vi "DDS_Clock.vi"() -> ()   [LabVIEW 2016] (continued)
{"total time[ms]"=60.64999999999869, "f1 [Hz] CH0"=302600000.00000006}, {"total time[ms]"=60.69999999999869, "f1 [Hz] CH0"=302800000.0}, {"total time[ms]"=60.69999999999869, "f1 [Hz] CH0"=302800000.0}, {"total time[ms]"=60.749999999998685, "f1 [Hz] CH0"=303000000.0}, {"total time[ms]"=60.749999999998685, "f1 [Hz] CH0"=303000000.0}, {"total time[ms]"=60.79999999999868, "f1 [Hz] CH0"=303200000.00000006}, {"total time[ms]"=60.79999999999868, "f1 [Hz] CH0"=303200000.00000006}, {"total time[ms]"=60.84999999999868, "f1 [Hz] CH0"=303400000.00000006}, {"total time[ms]"=60.84999999999868, "f1 [Hz] CH0"=303400000.00000006}, {"total time[ms]"=60.89999999999868, "f1 [Hz] CH0"=303600000.0}, {"total time[ms]"=60.89999999999868, "f1 [Hz] CH0"=303600000.0}, {"total time[ms]"=60.949999999998674, "f1 [Hz] CH0"=303800000.0}, {"total time[ms]"=60.949999999998674, "f1 [Hz] CH0"=303800000.0}, {"total time[ms]"=60.99999999999867, "f1 [Hz] CH0"=304000000.0}, {"total time[ms]"=60.99999999999867, "f1 [Hz] CH0"=304000000.0}, {"total time[ms]"=61.04999999999867, "f1 [Hz] CH0"=304200000.0}, {"total time[ms]"=61.04999999999867, "f1 [Hz] CH0"=304200000.0}, {"total time[ms]"=61.099999999998666, "f1 [Hz] CH0"=304400000.0}, {"total time[ms]"=61.099999999998666, "f1 [Hz] CH0"=304400000.0}, {"total time[ms]"=61.14999999999866, "f1 [Hz] CH0"=304600000.00000006}, {"total time[ms]"=61.14999999999866, "f1 [Hz] CH0"=304600000.00000006}, {"total time[ms]"=61.19999999999866, "f1 [Hz] CH0"=304800000.00000006}, {"total time[ms]"=61.19999999999866, "f1 [Hz] CH0"=304800000.00000006}, {"total time[ms]"=61.24999999999866, "f1 [Hz] CH0"=305000000.0}, {"total time[ms]"=61.24999999999866, "f1 [Hz] CH0"=305000000.0}, {"total time[ms]"=61.299999999998654, "f1 [Hz] CH0"=305200000.00000006}, {"total time[ms]"=61.299999999998654, "f1 [Hz] CH0"=305200000.00000006}, {"total time[ms]"=61.34999999999865, "f1 [Hz] CH0"=305400000.0}, {"total time[ms]"=61.34999999999865, "f1 [Hz] CH0"=305400000.0}, {"total time[ms]"=61.39999999999865, "f1 [Hz] CH0"=305600000.0}, {"total time[ms]"=61.39999999999865, "f1 [Hz] CH0"=305600000.0}, {"total time[ms]"=61.449999999998646, "f1 [Hz] CH0"=305800000.0}, {"total time[ms]"=61.449999999998646, "f1 [Hz] CH0"=305800000.0}, {"total time[ms]"=61.49999999999864, "f1 [Hz] CH0"=306000000.0}, {"total time[ms]"=61.49999999999864, "f1 [Hz] CH0"=306000000.0}, {"total time[ms]"=61.54999999999864, "f1 [Hz] CH0"=306200000.00000006}, {"total time[ms]"=61.54999999999864, "f1 [Hz] CH0"=306200000.00000006}, {"total time[ms]"=61.59999999999864, "f1 [Hz] CH0"=306400000.0}, {"total time[ms]"=61.59999999999864, "f1 [Hz] CH0"=306400000.0}, {"total time[ms]"=61.649999999998634, "f1 [Hz] CH0"=306600000.00000006}, {"total time[ms]"=61.649999999998634, "f1 [Hz] CH0"=306600000.00000006}, {"total time[ms]"=61.69999999999863, "f1 [Hz] CH0"=306800000.00000006}, {"total time[ms]"=61.69999999999863, "f1 [Hz] CH0"=306800000.00000006}, {"total time[ms]"=61.74999999999863, "f1 [Hz] CH0"=307000000.0}, {"total time[ms]"=61.74999999999863, "f1 [Hz] CH0"=307000000.0}, {"total time[ms]"=61.799999999998626, "f1 [Hz] CH0"=307200000.0}, {"total time[ms]"=61.799999999998626, "f1 [Hz] CH0"=307200000.0}, {"total time[ms]"=61.84999999999862, "f1 [Hz] CH0"=307400000.0}, {"total time[ms]"=61.84999999999862, "f1 [Hz] CH0"=307400000.0}, {"total time[ms]"=61.89999999999862, "f1 [Hz] CH0"=307600000.00000006}, {"total time[ms]"=61.89999999999862, "f1 [Hz] CH0"=307600000.00000006}, {"total time[ms]"=61.94999999999862, "f1 [Hz] CH0"=307800000.0}, {"total time[ms]"=61.94999999999862, "f1 [Hz] CH0"=307800000.0}, {"total time[ms]"=61.999999999998614, "f1 [Hz] CH0"=308000000.0}, {"total time[ms]"=61.999999999998614, "f1 [Hz] CH0"=308000000.0}, {"total time[ms]"=62.04999999999861, "f1 [Hz] CH0"=308200000.00000006}, {"total time[ms]"=62.04999999999861, "f1 [Hz] CH0"=308200000.00000006}, {"total time[ms]"=62.09999999999861, "f1 [Hz] CH0"=308400000.00000006}, {"total time[ms]"=62.09999999999861, "f1 [Hz] CH0"=308400000.00000006}, {"total time[ms]"=62.149999999998606, "f1 [Hz] CH0"=308600000.0}, {"total time[ms]"=62.149999999998606, "f1 [Hz] CH0"=308600000.0}, {"total time[ms]"=62.1999999999986, "f1 [Hz] CH0"=308800000.0}, {"total time[ms]"=62.1999999999986, "f1 [Hz] CH0"=308800000.0}, {"total time[ms]"=62.2499999999986, "f1 [Hz] CH0"=309000000.0}, {"total time[ms]"=62.2499999999986, "f1 [Hz] CH0"=309000000.0}, {"total time[ms]"=62.2999999999986, "f1 [Hz] CH0"=309200000.0}, {"total time[ms]"=62.2999999999986, "f1 [Hz] CH0"=309200000.0}, {"total time[ms]"=62.349999999998595, "f1 [Hz] CH0"=309400000.0}, {"total time[ms]"=62.349999999998595, "f1 [Hz] CH0"=309400000.0}, {"total time[ms]"=62.39999999999859, "f1 [Hz] CH0"=309600000.00000006}, {"total time[ms]"=62.39999999999859, "f1 [Hz] CH0"=309600000.00000006}, {"total time[ms]"=62.44999999999859, "f1 [Hz] CH0"=309800000.00000006}, {"total time[ms]"=62.44999999999859, "f1 [Hz] CH0"=309800000.00000006}, {"total time[ms]"=62.499999999998586, "f1 [Hz] CH0"=310000000.0}, {"total time[ms]"=62.499999999998586, "f1 [Hz] CH0"=310000000.0}, {"total time[ms]"=62.54999999999858, "f1 [Hz] CH0"=310200000.00000006}, {"total time[ms]"=62.54999999999858, "f1 [Hz] CH0"=310200000.00000006}, {"total time[ms]"=62.59999999999858, "f1 [Hz] CH0"=310400000.0}, {"total time[ms]"=62.59999999999858, "f1 [Hz] CH0"=310400000.0}, {"total time[ms]"=62.64999999999858, "f1 [Hz] CH0"=310600000.0}, {"total time[ms]"=62.64999999999858, "f1 [Hz] CH0"=310600000.0}, {"total time[ms]"=62.699999999998575, "f1 [Hz] CH0"=310800000.0}, {"total time[ms]"=62.699999999998575, "f1 [Hz] CH0"=310800000.0}, {"total time[ms]"=62.74999999999857, "f1 [Hz] CH0"=311000000.0}, {"total time[ms]"=62.74999999999857, "f1 [Hz] CH0"=311000000.0}, {"total time[ms]"=62.79999999999857, "f1 [Hz] CH0"=311200000.00000006}, {"total time[ms]"=62.79999999999857, "f1 [Hz] CH0"=311200000.00000006}, {"total time[ms]"=62.849999999998566, "f1 [Hz] CH0"=311400000.0}, {"total time[ms]"=62.849999999998566, "f1 [Hz] CH0"=311400000.0}, {"total time[ms]"=62.89999999999856, "f1 [Hz] CH0"=311600000.00000006}, {"total time[ms]"=62.89999999999856, "f1 [Hz] CH0"=311600000.00000006}, {"total time[ms]"=62.94999999999856, "f1 [Hz] CH0"=311800000.00000006}, {"total time[ms]"=62.94999999999856, "f1 [Hz] CH0"=311800000.00000006}, {"total time[ms]"=62.99999999999856, "f1 [Hz] CH0"=312000000.0}, {"total time[ms]"=62.99999999999856, "f1 [Hz] CH0"=312000000.0}, {"total time[ms]"=63.049999999998555, "f1 [Hz] CH0"=312200000.0}, {"total time[ms]"=63.049999999998555, "f1 [Hz] CH0"=312200000.0}, {"total time[ms]"=63.09999999999855, "f1 [Hz] CH0"=312400000.0}, {"total time[ms]"=63.09999999999855, "f1 [Hz] CH0"=312400000.0}, {"total time[ms]"=63.14999999999855, "f1 [Hz] CH0"=312600000.00000006}, {"total time[ms]"=63.14999999999855, "f1 [Hz] CH0"=312600000.00000006}, {"total time[ms]"=63.199999999998546, "f1 [Hz] CH0"=312800000.0}, {"total time[ms]"=63.199999999998546, "f1 [Hz] CH0"=312800000.0}, {"total time[ms]"=63.24999999999854, "f1 [Hz] CH0"=313000000.0}, {"total time[ms]"=63.24999999999854, "f1 [Hz] CH0"=313000000.0}, {"total time[ms]"=63.29999999999854, "f1 [Hz] CH0"=313200000.00000006}, {"total time[ms]"=63.29999999999854, "f1 [Hz] CH0"=313200000.00000006}, {"total time[ms]"=63.34999999999854, "f1 [Hz] CH0"=313400000.00000006}, {"total time[ms]"=63.34999999999854, "f1 [Hz] CH0"=313400000.00000006}, {"total time[ms]"=63.399999999998535, "f1 [Hz] CH0"=313600000.0}, {"total time[ms]"=63.399999999998535, "f1 [Hz] CH0"=313600000.0}, {"total time[ms]"=63.44999999999853, "f1 [Hz] CH0"=313800000.0}, {"total time[ms]"=63.44999999999853, "f1 [Hz] CH0"=313800000.0}, {"total time[ms]"=63.49999999999853, "f1 [Hz] CH0"=314000000.0}, {"total time[ms]"=63.49999999999853, "f1 [Hz] CH0"=314000000.0}, {"total time[ms]"=63.549999999998526, "f1 [Hz] CH0"=314200000.0}, {"total time[ms]"=63.549999999998526, "f1 [Hz] CH0"=314200000.0}, {"total time[ms]"=63.59999999999852, "f1 [Hz] CH0"=314400000.0}, {"total time[ms]"=63.59999999999852, "f1 [Hz] CH0"=314400000.0}, {"total time[ms]"=63.64999999999852, "f1 [Hz] CH0"=314600000.00000006}, {"total time[ms]"=63.64999999999852, "f1 [Hz] CH0"=314600000.00000006}, {"total time[ms]"=63.69999999999852, "f1 [Hz] CH0"=314800000.00000006}, {"total time[ms]"=63.69999999999852, "f1 [Hz] CH0"=314800000.00000006}, {"total time[ms]"=63.749999999998515, "f1 [Hz] CH0"=315000000.0}, {"total time[ms]"=63.749999999998515, "f1 [Hz] CH0"=315000000.0}, {"total time[ms]"=63.79999999999851, "f1 [Hz] CH0"=315200000.00000006}, {"total time[ms]"=63.79999999999851, "f1 [Hz] CH0"=315200000.00000006}, {"total time[ms]"=63.84999999999851, "f1 [Hz] CH0"=315400000.0}, {"total time[ms]"=63.84999999999851, "f1 [Hz] CH0"=315400000.0}, {"total time[ms]"=63.899999999998506, "f1 [Hz] CH0"=315600000.0}, {"total time[ms]"=63.899999999998506, "f1 [Hz] CH0"=315600000.0}, {"total time[ms]"=63.949999999998504, "f1 [Hz] CH0"=315800000.0}, {"total time[ms]"=63.949999999998504, "f1 [Hz] CH0"=315800000.0}, {"total time[ms]"=63.9999999999985, "f1 [Hz] CH0"=316000000.0}, {"total time[ms]"=63.9999999999985, "f1 [Hz] CH0"=316000000.0}, {"total time[ms]"=64.0499999999985, "f1 [Hz] CH0"=316200000.0}, {"total time[ms]"=64.0499999999985, "f1 [Hz] CH0"=316200000.0}, {"total time[ms]"=64.0999999999985, "f1 [Hz] CH0"=316400000.00000006}, {"total time[ms]"=64.0999999999985, "f1 [Hz] CH0"=316400000.00000006}, {"total time[ms]"=64.1499999999985, "f1 [Hz] CH0"=316600000.00000006}, {"total time[ms]"=64.1499999999985, "f1 [Hz] CH0"=316600000.00000006}, {"total time[ms]"=64.1999999999985, "f1 [Hz] CH0"=316800000.00000006}, {"total time[ms]"=64.1999999999985, "f1 [Hz] CH0"=316800000.00000006}, {"total time[ms]"=64.2499999999985, "f1 [Hz] CH0"=317000000.0}, {"total time[ms]"=64.2499999999985, "f1 [Hz] CH0"=317000000.0}, {"total time[ms]"=64.29999999999849, "f1 [Hz] CH0"=317200000.0}, {"total time[ms]"=64.29999999999849, "f1 [Hz] CH0"=317200000.0}, {"total time[ms]"=64.34999999999849, "f1 [Hz] CH0"=317400000.00000006}, {"total time[ms]"=64.34999999999849, "f1 [Hz] CH0"=317400000.00000006}, {"total time[ms]"=64.39999999999849, "f1 [Hz] CH0"=317600000.00000006}, {"total time[ms]"=64.39999999999849, "f1 [Hz] CH0"=317600000.00000006}, {"total time[ms]"=64.44999999999848, "f1 [Hz] CH0"=317800000.0}, {"total time[ms]"=64.44999999999848, "f1 [Hz] CH0"=317800000.0}, {"total time[ms]"=64.49999999999848, "f1 [Hz] CH0"=318000000.0}, {"total time[ms]"=64.49999999999848, "f1 [Hz] CH0"=318000000.0}, {"total time[ms]"=64.54999999999848, "f1 [Hz] CH0"=318200000.0}, {"total time[ms]"=64.54999999999848, "f1 [Hz] CH0"=318200000.0}, {"total time[ms]"=64.59999999999847, "f1 [Hz] CH0"=318400000.00000006}, {"total time[ms]"=64.59999999999847, "f1 [Hz] CH0"=318400000.00000006}, {"total time[ms]"=64.64999999999847, "f1 [Hz] CH0"=318600000.0}, {"total time[ms]"=64.64999999999847, "f1 [Hz] CH0"=318600000.0}, {"total time[ms]"=64.69999999999847, "f1 [Hz] CH0"=318800000.0}, {"total time[ms]"=64.69999999999847, "f1 [Hz] CH0"=318800000.0}, {"total time[ms]"=64.74999999999847, "f1 [Hz] CH0"=319000000.0}, {"total time[ms]"=64.74999999999847, "f1 [Hz] CH0"=319000000.0}, {"total time[ms]"=64.79999999999846, "f1 [Hz] CH0"=319200000.0}, {"total time[ms]"=64.79999999999846, "f1 [Hz] CH0"=319200000.0}, {"total time[ms]"=64.84999999999846, "f1 [Hz] CH0"=319400000.00000006}, {"total time[ms]"=64.84999999999846, "f1 [Hz] CH0"=319400000.00000006}, {"total time[ms]"=64.89999999999846, "f1 [Hz] CH0"=319600000.00000006}, {"total time[ms]"=64.89999999999846, "f1 [Hz] CH0"=319600000.00000006}, {"total time[ms]"=64.94999999999845, "f1 [Hz] CH0"=319800000.00000006}, {"total time[ms]"=64.94999999999845, "f1 [Hz] CH0"=319800000.00000006}, {"total time[ms]"=64.99999999999845, "f1 [Hz] CH0"=320000000.0}, {"total time[ms]"=64.99999999999845, "f1 [Hz] CH0"=320000000.0}, {"total time[ms]"=65.04999999999845, "f1 [Hz] CH0"=319800000.0}, {"total time[ms]"=65.04999999999845, "f1 [Hz] CH0"=319800000.0}, {"total time[ms]"=65.09999999999845, "f1 [Hz] CH0"=319599999.99999994}, {"total time[ms]"=65.09999999999845, "f1 [Hz] CH0"=319599999.99999994}, {"total time[ms]"=65.14999999999844, "f1 [Hz] CH0"=319400000.0}, {"total time[ms]"=65.14999999999844, "f1 [Hz] CH0"=319400000.0}, {"total time[ms]"=65.19999999999844, "f1 [Hz] CH0"=319200000.0}, {"total time[ms]"=65.19999999999844, "f1 [Hz] CH0"=319200000.0}, {"total time[ms]"=65.24999999999844, "f1 [Hz] CH0"=319000000.0}, {"total time[ms]"=65.24999999999844, "f1 [Hz] CH0"=319000000.0}, {"total time[ms]"=65.29999999999843, "f1 [Hz] CH0"=318800000.0}, {"total time[ms]"=65.29999999999843, "f1 [Hz] CH0"=318800000.0}, {"total time[ms]"=65.34999999999843, "f1 [Hz] CH0"=318599999.99999994}, {"total time[ms]"=65.34999999999843, "f1 [Hz] CH0"=318599999.99999994}, {"total time[ms]"=65.39999999999843, "f1 [Hz] CH0"=318399999.99999994}, {"total time[ms]"=65.39999999999843, "f1 [Hz] CH0"=318399999.99999994}, {"total time[ms]"=65.44999999999843, "f1 [Hz] CH0"=318199999.99999994}, {"total time[ms]"=65.44999999999843, "f1 [Hz] CH0"=318199999.99999994}, {"total time[ms]"=65.49999999999842, "f1 [Hz] CH0"=318000000.0}, {"total time[ms]"=65.49999999999842, "f1 [Hz] CH0"=318000000.0}, {"total time[ms]"=65.54999999999842, "f1 [Hz] CH0"=317800000.0}, {"total time[ms]"=65.54999999999842, "f1 [Hz] CH0"=317800000.0}, {"total time[ms]"=65.59999999999842, "f1 [Hz] CH0"=317599999.99999994}, {"total time[ms]"=65.59999999999842, "f1 [Hz] CH0"=317599999.99999994}, {"total time[ms]"=65.64999999999841, "f1 [Hz] CH0"=317399999.99999994}, {"total time[ms]"=65.64999999999841, "f1 [Hz] CH0"=317399999.99999994}, {"total time[ms]"=65.69999999999841, "f1 [Hz] CH0"=317200000.0}, {"total time[ms]"=65.69999999999841, "f1 [Hz] CH0"=317200000.0}, {"total time[ms]"=65.74999999999841, "f1 [Hz] CH0"=317000000.0}, {"total time[ms]"=65.74999999999841, "f1 [Hz] CH0"=317000000.0}, {"total time[ms]"=65.7999999999984, "f1 [Hz] CH0"=316800000.0}, {"total time[ms]"=65.7999999999984, "f1 [Hz] CH0"=316800000.0}, {"total time[ms]"=65.8499999999984, "f1 [Hz] CH0"=316599999.99999994}, {"total time[ms]"=65.8499999999984, "f1 [Hz] CH0"=316599999.99999994}, {"total time[ms]"=65.8999999999984, "f1 [Hz] CH0"=316400000.0}, {"total time[ms]"=65.8999999999984, "f1 [Hz] CH0"=316400000.0}, {"total time[ms]"=65.9499999999984, "f1 [Hz] CH0"=316200000.0}, {"total time[ms]"=65.9499999999984, "f1 [Hz] CH0"=316200000.0}, {"total time[ms]"=65.9999999999984, "f1 [Hz] CH0"=316000000.0}, {"total time[ms]"=65.9999999999984, "f1 [Hz] CH0"=316000000.0}, {"total time[ms]"=66.04999999999839, "f1 [Hz] CH0"=315800000.0}, {"total time[ms]"=66.04999999999839, "f1 [Hz] CH0"=315800000.0}, {"total time[ms]"=66.09999999999839, "f1 [Hz] CH0"=315599999.99999994}, {"total time[ms]"=66.09999999999839, "f1 [Hz] CH0"=315599999.99999994}, {"total time[ms]"=66.14999999999839, "f1 [Hz] CH0"=315399999.99999994}, {"total time[ms]"=66.14999999999839, "f1 [Hz] CH0"=315399999.99999994}, {"total time[ms]"=66.19999999999838, "f1 [Hz] CH0"=315199999.99999994}, {"total time[ms]"=66.19999999999838, "f1 [Hz] CH0"=315199999.99999994}, {"total time[ms]"=66.24999999999838, "f1 [Hz] CH0"=315000000.0}, {"total time[ms]"=66.24999999999838, "f1 [Hz] CH0"=315000000.0}, {"total time[ms]"=66.29999999999838, "f1 [Hz] CH0"=314800000.0}, {"total time[ms]"=66.29999999999838, "f1 [Hz] CH0"=314800000.0}, {"total time[ms]"=66.34999999999837, "f1 [Hz] CH0"=314599999.99999994}, {"total time[ms]"=66.34999999999837, "f1 [Hz] CH0"=314599999.99999994}, {"total time[ms]"=66.39999999999837, "f1 [Hz] CH0"=314400000.0}, {"total time[ms]"=66.39999999999837, "f1 [Hz] CH0"=314400000.0}, {"total time[ms]"=66.44999999999837, "f1 [Hz] CH0"=314200000.0}, {"total time[ms]"=66.44999999999837, "f1 [Hz] CH0"=314200000.0}, {"total time[ms]"=66.49999999999837, "f1 [Hz] CH0"=314000000.0}, {"total time[ms]"=66.49999999999837, "f1 [Hz] CH0"=314000000.0}, {"total time[ms]"=66.54999999999836, "f1 [Hz] CH0"=313800000.0}, {"total time[ms]"=66.54999999999836, "f1 [Hz] CH0"=313800000.0}, {"total time[ms]"=66.59999999999836, "f1 [Hz] CH0"=313599999.99999994}, {"total time[ms]"=66.59999999999836, "f1 [Hz] CH0"=313599999.99999994}, {"total time[ms]"=66.64999999999836, "f1 [Hz] CH0"=313399999.99999994}, {"total time[ms]"=66.64999999999836, "f1 [Hz] CH0"=313399999.99999994}, {"total time[ms]"=66.69999999999835, "f1 [Hz] CH0"=313199999.99999994}, {"total time[ms]"=66.69999999999835, "f1 [Hz] CH0"=313199999.99999994}, {"total time[ms]"=66.74999999999835, "f1 [Hz] CH0"=313000000.0}, {"total time[ms]"=66.74999999999835, "f1 [Hz] CH0"=313000000.0}, {"total time[ms]"=66.79999999999835, "f1 [Hz] CH0"=312800000.0}, {"total time[ms]"=66.79999999999835, "f1 [Hz] CH0"=312800000.0}, {"total time[ms]"=66.84999999999835, "f1 [Hz] CH0"=312599999.99999994}, {"total time[ms]"=66.84999999999835, "f1 [Hz] CH0"=312599999.99999994}, {"total time[ms]"=66.89999999999834, "f1 [Hz] CH0"=312399999.99999994}, {"total time[ms]"=66.89999999999834, "f1 [Hz] CH0"=312399999.99999994}, {"total time[ms]"=66.94999999999834, "f1 [Hz] CH0"=312200000.0}, {"total time[ms]"=66.94999999999834, "f1 [Hz] CH0"=312200000.0}, {"total time[ms]"=66.99999999999834, "f1 [Hz] CH0"=312000000.0}, {"total time[ms]"=66.99999999999834, "f1 [Hz] CH0"=312000000.0}, {"total time[ms]"=67.04999999999833, "f1 [Hz] CH0"=311800000.0}, {"total time[ms]"=67.04999999999833, "f1 [Hz] CH0"=311800000.0}, {"total time[ms]"=67.09999999999833, "f1 [Hz] CH0"=311599999.99999994}, {"total time[ms]"=67.09999999999833, "f1 [Hz] CH0"=311599999.99999994}, {"total time[ms]"=67.14999999999833, "f1 [Hz] CH0"=311400000.0}, {"total time[ms]"=67.14999999999833, "f1 [Hz] CH0"=311400000.0}, {"total time[ms]"=67.19999999999833, "f1 [Hz] CH0"=311200000.0}, {"total time[ms]"=67.19999999999833, "f1 [Hz] CH0"=311200000.0}, {"total time[ms]"=67.24999999999832, "f1 [Hz] CH0"=311000000.0}, {"total time[ms]"=67.24999999999832, "f1 [Hz] CH0"=311000000.0}, {"total time[ms]"=67.29999999999832, "f1 [Hz] CH0"=310800000.0}, {"total time[ms]"=67.29999999999832, "f1 [Hz] CH0"=310800000.0}, {"total time[ms]"=67.34999999999832, "f1 [Hz] CH0"=310599999.99999994}, {"total time[ms]"=67.34999999999832, "f1 [Hz] CH0"=310599999.99999994}, {"total time[ms]"=67.39999999999831, "f1 [Hz] CH0"=310399999.99999994}, {"total time[ms]"=67.39999999999831, "f1 [Hz] CH0"=310399999.99999994}, {"total time[ms]"=67.44999999999831, "f1 [Hz] CH0"=310199999.99999994}, {"total time[ms]"=67.44999999999831, "f1 [Hz] CH0"=310199999.99999994}, {"total time[ms]"=67.49999999999831, "f1 [Hz] CH0"=310000000.0}, {"total time[ms]"=67.49999999999831, "f1 [Hz] CH0"=310000000.0}, {"total time[ms]"=67.5499999999983, "f1 [Hz] CH0"=309800000.0}, {"total time[ms]"=67.5499999999983, "f1 [Hz] CH0"=309800000.0}, {"total time[ms]"=67.5999999999983, "f1 [Hz] CH0"=309599999.99999994}, {"total time[ms]"=67.5999999999983, "f1 [Hz] CH0"=309599999.99999994}, {"total time[ms]"=67.6499999999983, "f1 [Hz] CH0"=309400000.0}, {"total time[ms]"=67.6499999999983, "f1 [Hz] CH0"=309400000.0}, {"total time[ms]"=67.6999999999983, "f1 [Hz] CH0"=309200000.0}, {"total time[ms]"=67.6999999999983, "f1 [Hz] CH0"=309200000.0}, {"total time[ms]"=67.7499999999983, "f1 [Hz] CH0"=309000000.0}, {"total time[ms]"=67.7499999999983, "f1 [Hz] CH0"=309000000.0}, {"total time[ms]"=67.79999999999829, "f1 [Hz] CH0"=308800000.0}, {"total time[ms]"=67.79999999999829, "f1 [Hz] CH0"=308800000.0}, {"total time[ms]"=67.84999999999829, "f1 [Hz] CH0"=308599999.99999994}, {"total time[ms]"=67.84999999999829, "f1 [Hz] CH0"=308599999.99999994}, {"total time[ms]"=67.89999999999829, "f1 [Hz] CH0"=308399999.99999994}, {"total time[ms]"=67.89999999999829, "f1 [Hz] CH0"=308399999.99999994}, {"total time[ms]"=67.94999999999828, "f1 [Hz] CH0"=308199999.99999994}, {"total time[ms]"=67.94999999999828, "f1 [Hz] CH0"=308199999.99999994}, {"total time[ms]"=67.99999999999828, "f1 [Hz] CH0"=308000000.0}, {"total time[ms]"=67.99999999999828, "f1 [Hz] CH0"=308000000.0}, {"total time[ms]"=68.04999999999828, 
